vi "GetText.vi"(8 "error in":errorcluster, 11 "Polynomial Scale editor node in":refnum<class "Polynomial Scale editor node.lvclass">) -> (0 "error out":errorcluster, 1 "additional text":string, 2 "text":string, 3 "Polynomial Scale editor node out":refnum<class "Polynomial Scale editor node.lvclass">, 4 "glyph":string)   [LabVIEW 2013, in "Polynomial Scale editor node.lvclass"]
uses:
  Polynomial Scale editor node.lvclass
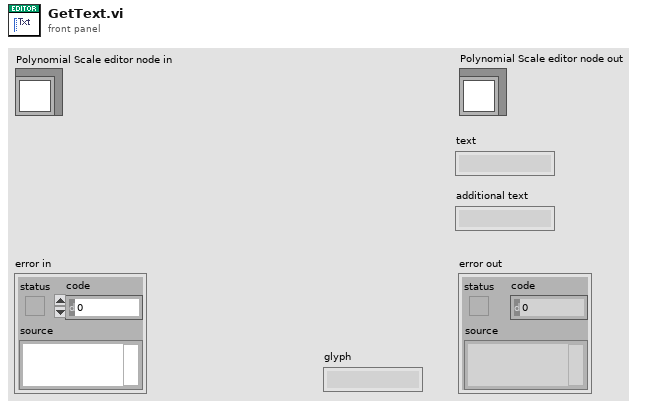
[diagram p1: front panel]
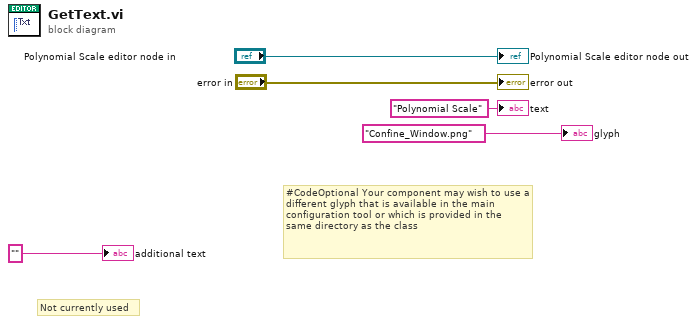
[diagram p0: block diagram]
diagram:
  # "Not currently used"
  # "#CodeOptional Your component may wish to use a different glyph that is available in the main configuration tool or which is provided in the same directory as the class"
  "error out" <- "error in"
  "Polynomial Scale editor node out" <- "Polynomial Scale editor node in"
  "text" <- "Polynomial Scale" ("text")
  "additional text" <- "" ("additional text")
  "glyph" <- "Confine_Window.png" ("glyph")
